vi "4_Sine Signal.vi"() -> ()   [LabVIEW 2018]
panel:
  in  "stop":bool
  out "Waveform Graph":dynamicdata(graph)
  in  "Frequency":dbl(knob) scale=0.0..10.0
  in  "Amplitude":dbl(knob) scale=0.0..10.0
  # "HMI Code for Sine Signal"
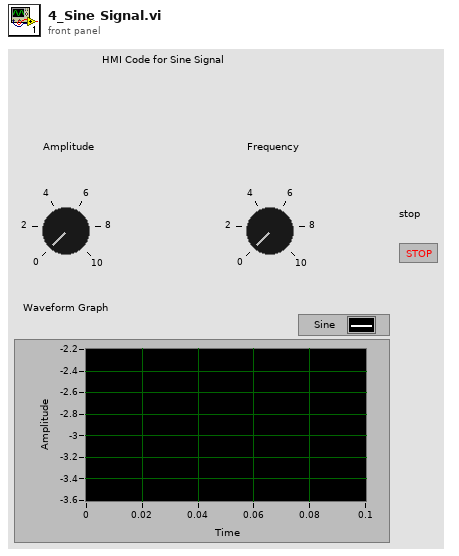
[diagram p1: front panel]
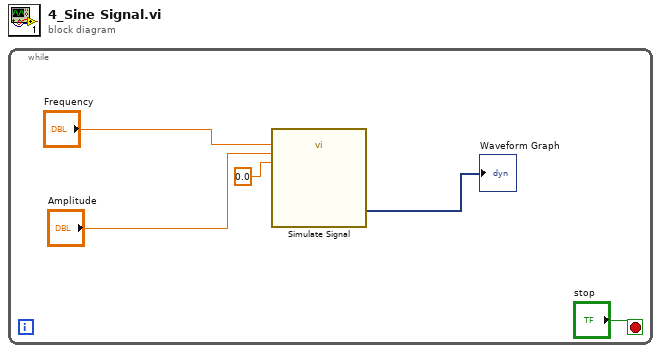
[diagram p0: block diagram]
diagram:
  n1 = while {
    stop <- "stop" stop-if-true
    n2 = call "Simulate Signal"("Frequency"="Frequency", "Amplitude"="Amplitude", "Phase"=0.0) -> ("Sine"=→"Waveform Graph":dynamicdata)  [unwired: 11 in, 1 out]
  }
